vi "Instr_InitObject.vi"(8 "error in (no error)":errorcluster, 9 "Instrument Configuration":variant, 10 "GPIB address":string, 11 "SupplyControl in":refnum<class "SupplyControl.lvclass">) -> (0 "error out":errorcluster, 3 "SupplyControl out":refnum<class "SupplyControl.lvclass">)   [LabVIEW 2018, in "SupplyControl.lvclass"]
uses:
  SupplyControl.lvclass
  InstrControl.lvclass
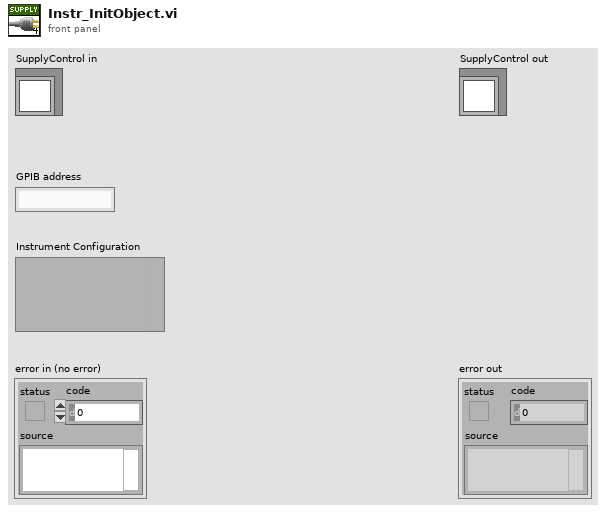
[diagram p1: front panel]
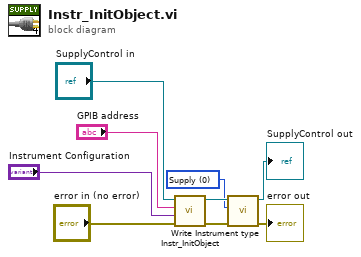
[diagram p0: block diagram]
diagram:
  w2 = u16 0 items=["Supply", "LCR", "Switching", "Multimeter"] ("Instrument type")
  n1 = call-parent "Instr_InitObject.vi"("error in (no error)"="error in (no error)", "Instrument Configuration"="Instrument Configuration", "GPIB Address"="GPIB address", "InstrControl in"="SupplyControl in") -> ("error out"=w5:errorcluster, "InstrControl out"=w6:refnum<class "SupplyControl.lvclass">)  [unwired: 6 in]
  n2 = call-dynamic "Write Instrument type.vi"("error in (no error)"=w5, "Instrument type"=w2, "InstControl in"=w6) -> ("error out"=→"error out":errorcluster, "InstControl out"=→"SupplyControl out":refnum<class "SupplyControl.lvclass">)  [unwired: 7 in]
